vi "subRetrieveAccelValues.vi"(2 "error in":errorcluster, 3 "AccelState":refnum<k24>, 4 "WiimoteState":refnum<k24>) -> (0 "error out":errorcluster, 1 "Wiimote State":T1)   [LabVIEW 2011]
uses:
  C:/Users/Nikos/Desktop/RTDSP PROJECT/Project RTDSP V16_TEST/Project RTDSP/rtdsp_project/3D_Experiment/libs/experiments 2/Resources/WiimoteLib.dll
  Project RTDSP V16_TEST/Project RTDSP/rtdsp_project/3D_Experiment/libs/experiments 2/Resources/WiimoteLib.dll
  Custom Controls/WiimoteState.ctl
panel:
  # "Accelerometers"
  # "Buttons"
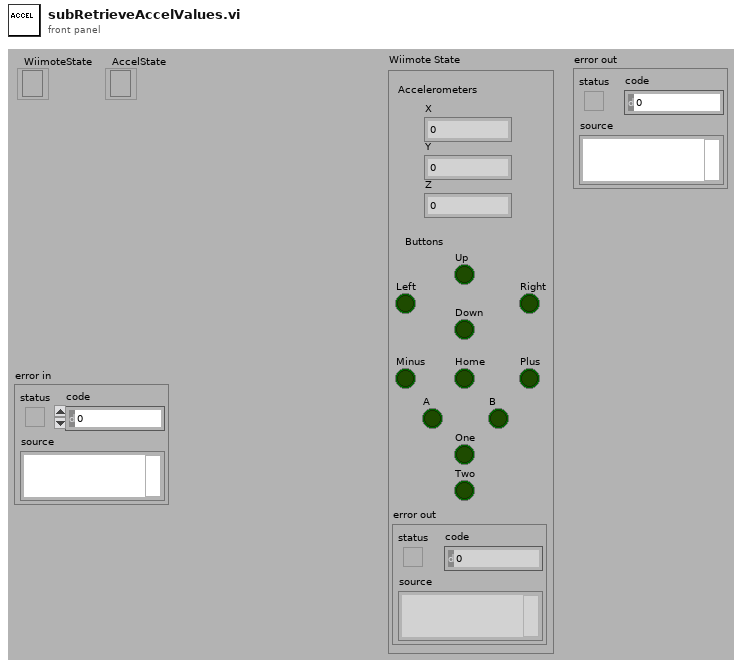
[diagram p1: front panel]
types:
  T1 = typedef "wiimotestate.ctl" = cluster{"X":sgl, "Y":sgl, "Z":sgl, "A":bool, "B":bool, "Down":bool, "Home":bool, "Left":bool, "Minus":bool, "One":bool, "Plus":bool, "Right":bool, "Two":bool, "Up":bool, "error out":errorcluster}
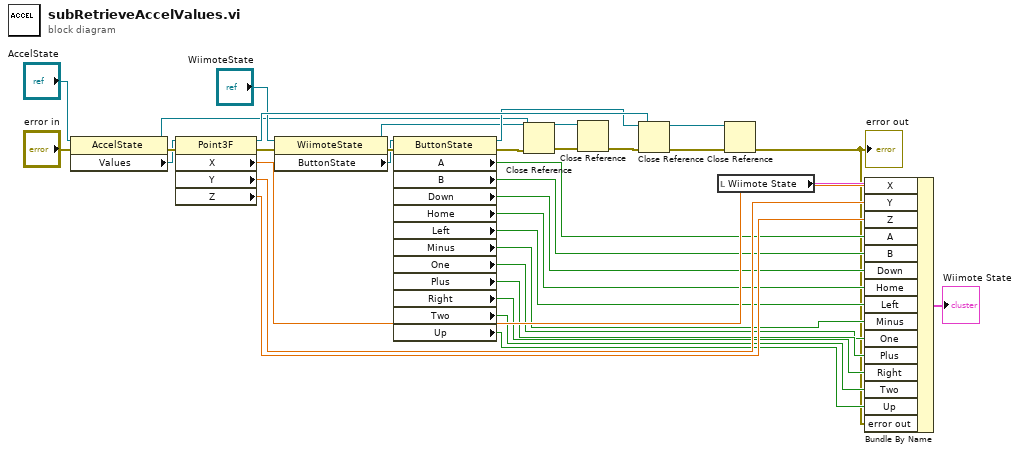
[diagram p0: block diagram]
diagram:
  n1 = property class="AccelState"(reference="AccelState", error in="error in") -> (reference out=w5:refnum<k24>, error out=w30:errorcluster, "Values"=w22:refnum<k24>)
  n2 = property class="Point3F"(reference=w22, error in=w30) -> (reference out=w31:refnum<k24>, error out=w33:errorcluster, "X"=w23:sgl, "Y"=w24:sgl, "Z"=w25:sgl)
  n3 = property class="WiimoteState"(reference="WiimoteState", error in=w33) -> (reference out=w3:refnum<k24>, error out=w28:errorcluster, "ButtonState"=w27:refnum<k24>)
  n4 = property class="ButtonState"(reference=w27, error in=w28) -> (reference out=w29:refnum<k24>, error out=w4:errorcluster, "A"=w10:bool, "B"=w11:bool, "Down"=w12:bool, "Home"=w13:bool, "Left"=w14:bool, "Minus"=w15:bool, "One"=w16:bool, "Plus"=w17:bool, "Right"=w18:bool, "Two"=w19:bool, "Up"=w20:bool)
  n5 = Close Reference(reference=w5, error in (no error)=w4) -> (error out=w2:errorcluster)
  n6 = Close Reference(reference=w3, error in (no error)=w2) -> (error out=w1:errorcluster)
  n7 = Close Reference(reference=w29, error in (no error)=w1) -> (error out=w6:errorcluster)
  n8 = local read "Wiimote State"() -> (w8:T1)
  n9 = Close Reference(reference=w31, error in (no error)=w6) -> (error out=w7:errorcluster)
  "error out" <- w7
  n10 = Bundle By Name(cluster=w8, "X"=w23, "Y"=w24, "Z"=w25, "A"=w10, "B"=w11, "Down"=w12, "Home"=w13, "Left"=w14, "Minus"=w15, "One"=w16, "Plus"=w17, "Right"=w18, "Two"=w19, "Up"=w20, "error out"=w7) -> (→"Wiimote State":T1)
